vi "readFromXML.vi"(8 "error in (no error)":errorcluster, 10 "XML in":string="<Azimuth>\n  <degreesArc>44.33</degreesArc>\n  <minutesArc>33.22</minutesArc>\n  <secondsArc>22.11</secondsArc>\n</Azimuth>", 11 "Azimuth in":refnum<class "Azimuth.lvclass">) -> (0 "error out":errorcluster, 3 "Azimuth out":refnum<class "Azimuth.lvclass">)   [LabVIEW 2014, in "TCSDataDefinitions.lvlib" / "TCSCommand.lvlib" / "TargetConfiguration.lvlib" / "Target.lvlib" / "FixedTarget.lvlib" / "Azimuth.lvclass"]
uses:
  Azimuth.lvclass
  <userlib>/Common/UnitsAndXML/FlattenItemWithUnitToXML/FlattenPlaneAngleToXML/PlaneAngleUnit.ctl
  Azimuth.lvclass/Azimuth.ctl
  <userlib>/Common/UnitsAndXML/UnitsAndXML.lvlib
  <userlib>/Common/XML/XMLParser/XMLParser.lvclass
panel:
  out "secondsArc":dbl[unit]=0.00010719230489331841
  out "minutesArc":dbl[unit]=0.00966330629187527
  out "degreesArc":dbl[unit]=0.7737044574090862
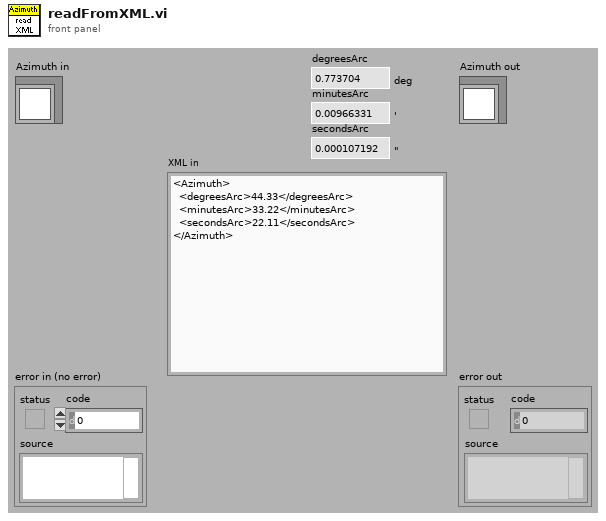
[diagram p1: front panel]
types:
  T1 = typedef "UnitsAndXML.lvlib/PlaneAngleUnit.ctl" = enum16{"rad", "deg", "'", "\""}
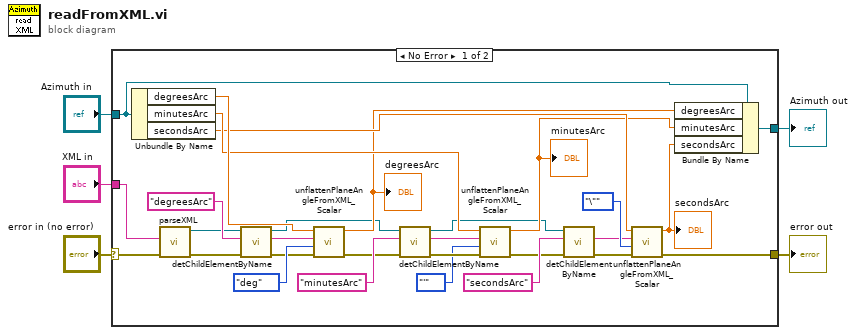
[diagram p0: block diagram]
diagram:
  n1 = case shown="No Error" "error in (no error)" {
    selector: "error in (no error)" -> [w33 w36]
    tunnel: [w18 w36] -> w4
    tunnel: [w30 w35] -> w2
    tunnel: "Azimuth in" -> [w31 w35]
    tunnel: "XML in" -> [w34 _]
    frame No Error {
      n2 = Unbundle By Name(w31) -> ("degreesArc"=w26:dbl[unit], "minutesArc"=w13:dbl[unit], "secondsArc"=w12:dbl[unit])
      n3 = call <userlib>:"parseXML.vi"("error in (no error)"=w33, "XMLString in"=w34) -> ("error out"=w32:errorcluster, "Element out"=w8:refnum<class "XMLParser.lvclass">)  [unwired: 8 in]
      n4 = call <userlib>:"detChildElementByName.vi"("error in (no error)"=w32, "childName"="degreesArc" ("ChildName"), "Element in"=w8) -> ("error out"=w23:errorcluster, "childXML"=w25:string, "Element out"=w7:refnum<class "XMLParser.lvclass">)  [unwired: 5 in, 1 out]
      n5 = call <userlib>:"unflattenPlaneAngleFromXML_Scalar.vi"("error in (no error)"=w23, "planeAngleUnitInXML"=PlaneAngleUnit."deg", "xmlString"=w25, "planeAngleForType"=w26) -> ("error out"=w22:errorcluster, "planeAngle"=w10:dbl[unit])  [unwired: 6 in]
      "degreesArc" <- w10
      n6 = call <userlib>:"detChildElementByName.vi"("error in (no error)"=w22, "childName"="minutesArc" ("ChildName"), "Element in"=w7) -> ("error out"=w21:errorcluster, "childXML"=w14:string, "Element out"=w6:refnum<class "XMLParser.lvclass">)  [unwired: 5 in, 1 out]
      n7 = call <userlib>:"unflattenPlaneAngleFromXML_Scalar.vi"("error in (no error)"=w21, "planeAngleUnitInXML"=PlaneAngleUnit."'", "xmlString"=w14, "planeAngleForType"=w13) -> ("error out"=w20:errorcluster, "planeAngle"=w11:dbl[unit])  [unwired: 6 in]
      "minutesArc" <- w11
      n8 = call <userlib>:"detChildElementByName.vi"("error in (no error)"=w20, "childName"="secondsArc" ("ChildName"), "Element in"=w6) -> ("error out"=w19:errorcluster, "childXML"=w15:string)  [unwired: 5 in, 2 out]
      n9 = call <userlib>:"unflattenPlaneAngleFromXML_Scalar.vi"("error in (no error)"=w19, "planeAngleUnitInXML"=PlaneAngleUnit."\"", "xmlString"=w15, "planeAngleForType"=w12) -> ("error out"=w18:errorcluster, "planeAngle"=w9:dbl[unit])  [unwired: 6 in]
      "secondsArc" <- w9
      n10 = Bundle By Name(cluster=w31, "degreesArc"=w10, "minutesArc"=w11, "secondsArc"=w9) -> (w30:refnum<class "Azimuth.lvclass">)
    }
    frame Error {
    }
  }
  "error out" <- w4
  "Azimuth out" <- w2
